vi "Write Scale Visible.vi"(8 "error in (no error)":errorcluster, 9 "Visible":bool, 10 "Y Scale Index":i32, 11 "Chart in":refnum<vi>) -> (0 "error out":errorcluster, 3 "Chart":refnum<vi>)   [LabVIEW 2020, in "VolatusGUIEditorCore.lvlib"]
uses:
  VolatusGUIEditorCore.lvlib
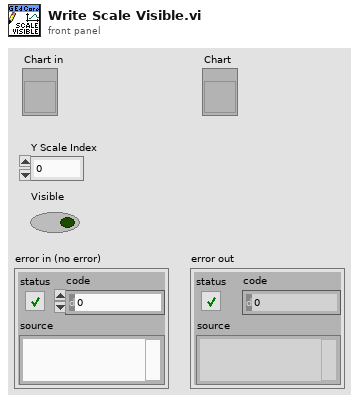
[diagram p1: front panel]
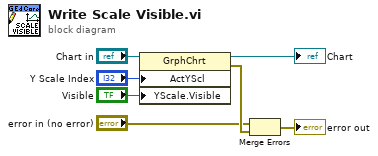
[diagram p0: block diagram]
diagram:
  n1 = property class="GrphChrt"(reference="Chart in", "ActYScl"="Y Scale Index", "YScale.Visible"="Visible") -> (reference out=→"Chart":refnum<vi>, error out=w3:errorcluster)  [unwired: 1 in]
  n2 = Merge Errors("error in (no error)", w3) -> (→"error out":errorcluster)
